vi "Ismatec 4083 Test Program Copy.vi"() -> ()   [LabVIEW 2021, in "Ismatec 4308.lvlib"]
uses:
  Ismatec 4308.lvlib
  Ismatec 4083.ctl
panel:
  out "No Pump Connected":bool=TRUE
  out "Initialized":bool
  out "Ismatech 3 Channel Settings Out":T1={"VISA resource name"="", "Pump Number"=1, "Channel Number"=0, "Simulated?"=TRUE, "Reverse?"=FALSE} {"Channel Number" min=0 max=3; "Pump Number" min=1 max=9}
  in  "Ismatech 3 Channel Settings In":T1={"VISA resource name"="COM5", "Pump Number"=6, "Channel Number"=2, "Simulated?"=FALSE, "Reverse?"=FALSE} {"Channel Number" min=0 max=3; "Pump Number" min=1 max=9}
  out "error out":errorcluster
  in  "error in (no error)":errorcluster
  in  "Speed (%)":dbl
  in  "Pause":bool
  out "Connection Error":bool
  out "Pump On?":enum16{"Off", "On", "Not Initialized"}(ring)
  out "Connection Error 2":bool
  in  "stop":bool
  out "error out 2":errorcluster
  out "error out 3":errorcluster
  out "RPM":dbl
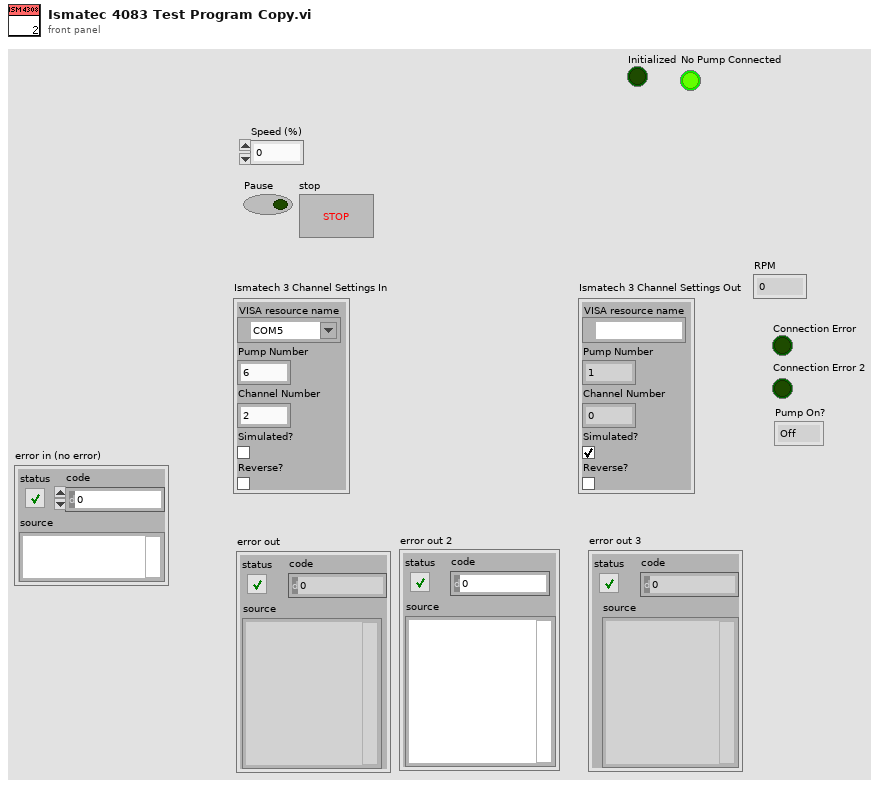
[diagram p1: front panel]
types:
  T1 = typedef "Ismatec 4308.lvlib/Ismatec 4083.ctl" = cluster{"VISA resource name":refnum<visa-resource-name>, "Pump Number":i16, "Channel Number":i16, "Simulated?":bool, "Reverse?":bool}
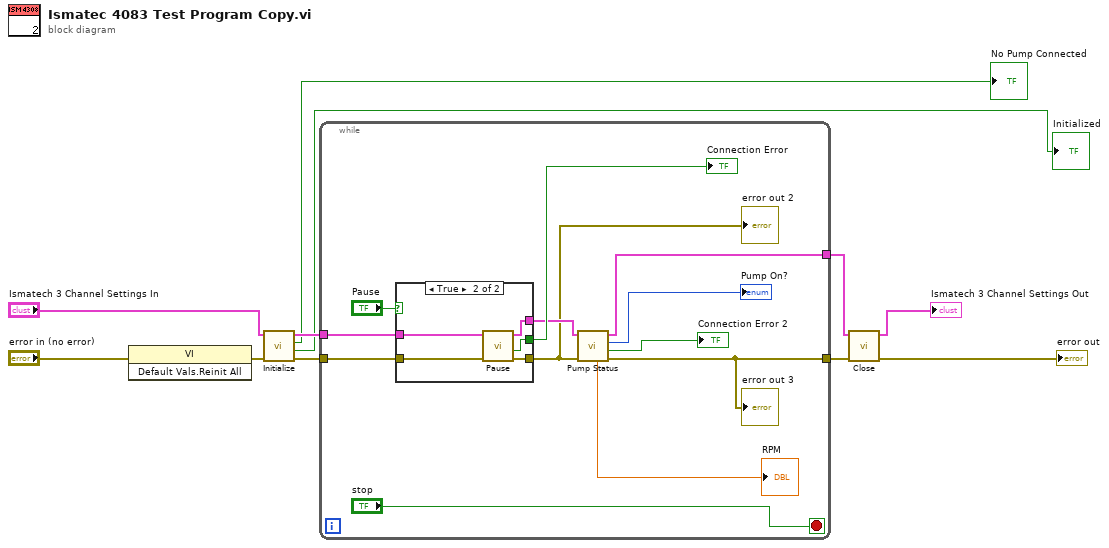
[diagram p0: block diagram]
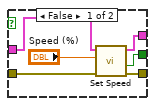
[diagram p2: hidden frame]
diagram:
  n1 = invoke class="VI" method="Default Vals.Reinit All"(error in="error in (no error)") -> (error out=w1:errorcluster)  [unwired: 2 in, 2 out]
  n2 = call "Initialize.vi"("error in (no error)"=w1, "Ismatech 3 Channel Settings In"="Ismatech 3 Channel Settings In") -> ("error out"=w9:errorcluster, "Initialized"=→"Initialized":bool, "No Pump Connected"=→"No Pump Connected":bool, "Ismatech 3 Channel Settings Out"=w10:T1)  [unwired: 6 in]
  n3 = while {
    tunnel: w10 -> [w22]
    tunnel: w9 -> [w21]
    tunnel: [w16] -> w8
    tunnel: [w13] -> w7
    stop <- "stop" stop-if-true
    n4 = case shown="True" "Pause" {
      tunnel: w22 -> [w28 w30]
      tunnel: w21 -> [w27 w31]
      tunnel: [w26 w33] -> w18
      tunnel: [w24 w32] -> w17
      tunnel: [w25 w34] -> w20
      frame False {
        n5 = call "Set Speed.vi"("error in (no error)"=w27, "Speed (%)"="Speed (%)", "Ismatech 3 Channel Settings In"=w28) -> ("error out"=w24:errorcluster, "Connection Error"=w25:bool, "Ismatech 3 Channel Settings Out"=w26:T1)  [unwired: 5 in, 1 out]
      }
      frame True {
        n6 = call "Pause.vi"("error in (no error)"=w31, "Ismatech 3 Channel Settings In"=w30) -> ("error out"=w32:errorcluster, "Connection Error"=w34:bool, "Ismatech 3 Channel Settings Out"=w33:T1)  [unwired: 6 in, 1 out]
      }
    }
    "Connection Error" <- w20
    "error out 2" <- w17
    n7 = call "Pump Status.vi"("error in (no error)"=w17, "Ismatech 3 Channel Settings In"=w18) -> ("error out"=w13:errorcluster, "Connection Error"=→"Connection Error 2":bool, "Pump On?"=→"Pump On?":enum16{"Off", "On", "Not Initialized"}, "Ismatech 3 Channel Settings Out"=w16:T1, "RPM"=→"RPM":dbl)  [unwired: 5 in]
    "error out 3" <- w13
  }
  n8 = call "Close.vi"("error in (no error)"=w7, "Ismatech 3 Channel Settings In"=w8) -> ("error out"=→"error out":errorcluster, "Ismatech 3 Channel Settings Out"=→"Ismatech 3 Channel Settings Out":T1)  [unwired: 7 in, 1 out]
